vi "FT_Close_Device.vi"(2 "error in":errorcluster, 3 "Handle":u32) -> (0 "error out":errorcluster, 1 "Handle out":u32)   [LabVIEW 2016]
uses:
  FTD2XX.dll
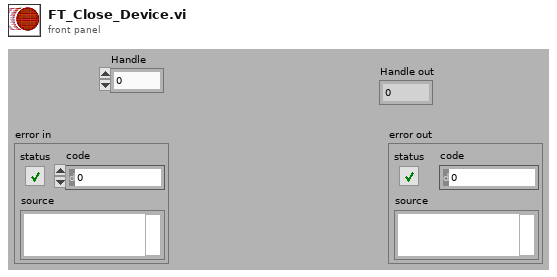
[diagram p1: front panel]
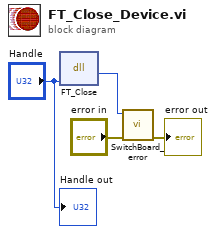
[diagram p0: block diagram]
diagram:
  n1 = dll-call lib="FTD2XX.dll" fn="FT_Close"("Handle"="Handle") -> ("FT_Status"=w1:u32)  [unwired: 4 in, 2 out]
  n2 = call "SwitchBoard_error.vi"("error constant"="error in", "Code"=w1) -> ("error IO"=→"error out":errorcluster)  [unwired: 9 in]
  "Handle out" <- "Handle"
